vi "prepareHeartbeat.vi"(8 "error in (no error)":errorcluster, 11 "DataListenerThisComponent in":refnum<class "DataListenerThisComponent.lvclass">) -> (0 "error out":errorcluster, 3 "DataListenerThisComponent out":refnum<class "DataListenerThisComponent.lvclass">)   [LabVIEW 2016, in "DataListenerThisComponent.lvclass"]
uses:
  DataListenerThisComponent.lvclass
  home/andres/ct_cmpuserevents/ComponentTemplateCore/ComponentModel/ComponentModel/DataListener/DataListener.lvclass
  ConfigurationTC/ConfigurationTypedefs/Base/HeartbeatConfig.ctl
  ConfigurationTC/ConfigurationTypedefs/ConfigurationTypedefs.lvlib
  ComponentTemplateCore/ComponentModel/ComponentModel/DataListener/DataListener.lvclass
  ComponentTemplateCore/ComponentModel/ComponentModel/ConfigurationFileReader/ConfigurationFileReader.lvclass
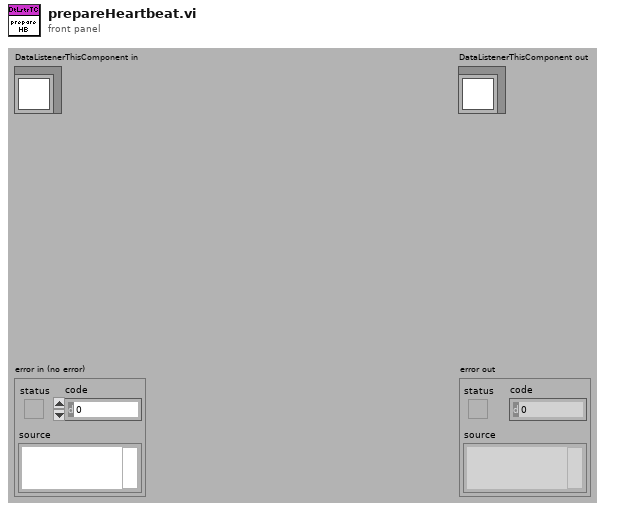
[diagram p1: front panel]
types:
  T1 = typedef "ConfigurationTypedefs.lvlib/HeartbeatConfig.ctl" = cluster{"Heartbeat Interval (s)":dbl, "Heartbeat Timeout (s)":dbl}
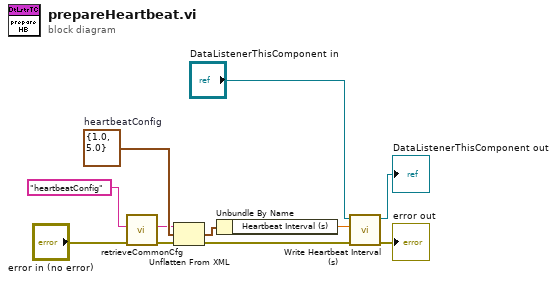
[diagram p0: block diagram]
diagram:
  w11 = T1 {"Heartbeat Interval (s)"=1.0, "Heartbeat Timeout (s)"=5.0}  # heartbeatConfig
  n1 = call "retrieveCommonCfg.vi"("error in (no error)"="error in (no error)", "dataName"="heartbeatConfig") -> ("error out"=w3:errorcluster, "dataValueFromFile"=w2:string)  [unwired: 7 in, 1 out]
  n2 = Unflatten From XML(xml string=w2, type=w11, error in (no error)=w3) -> (value=w10:T1, error out=w5:errorcluster)
  n3 = Unbundle By Name(w10) -> ("Heartbeat Interval (s)"=w9:dbl)
  n4 = call "Write Heartbeat Interval (s).vi"("error in (no error)"=w5, "Heartbeat Interval (s)"=w9, "DataListener in"="DataListenerThisComponent in") -> ("error out"=→"error out":errorcluster, "DataListener out"=→"DataListenerThisComponent out":refnum<class "DataListenerThisComponent.lvclass">)  [unwired: 7 in]
